vi "PID_Tuning.vi"() -> ()   [LabVIEW 2016]
uses:
  Classes/MotorControl/TypeDef/ControllerMode.ctl
  Classes/MotorControl/TypeDef/MotorTuneParam.ctl
  Classes/MotorControl/TypeDef/PID Param.ctl
  Classes/MotorControl/MotorControl.lvclass
  Classes/MotorControl/MotorControl.lvclass/MotorControl.ctl
  Classes/DataLogger/Data Logger.lvclass
  <vilib>/Platform/TimedLoop/XDataNode/timing_clust.ctl
  <vilib>/Platform/TimedLoop/XDataNode/nitl_modes.ctl
  <vilib>/Platform/TimedLoop/XDataNode/wakeup.ctl
  Classes/MotorControl/PropertyNodes/Motor_Read_Nx0.vi
  <vilib>/DAQmx/write.llb/DAQmx Write (Digital Bool 1Line 1Point).vi
  <vilib>/DAQmx/read.llb/DAQmx Read (Analog 1D Wfm NChan NSamp).vi
  <vilib>/Analysis/baseanly.llb/Mean (DBL).vi
  <vilib>/DAQmx/read.llb/DAQmx Read (Counter DBL 1Chan 1Samp).vi
  <vilib>/DAQmx/create/channels.llb/DAQmx Create Channel (CI-Position-Angular Encoder).vi
  <vilib>/FPGAPlugInAG/PXI-7842R/niLvFpga_Open_PXI-7842R.vi
  <vilib>/rvi/interface/common/dynamic/niFpgaDynamicAddResources.vi
  <vilib>/FPGAPlugInAG/Dynamic/niLvFpga_Reset_Dynamic.vi
  <vilib>/FPGAPlugInAG/Dynamic/niLvFpga_Run_Dynamic.vi
  <vilib>/Utility/error.llb/Error Cluster From Error Code.vi
  <vilib>/rvi/errors/niLvFpgaAdjustHostInterfaceError.vi
  GlobalVariables/Path_GV.vi
  <vilib>/DAQmx/miscellaneous.llb/DAQmx Fill In Error Info.vi
  <vilib>/measure/macond.llb/IIR Filter for N Chan.vi
  <vilib>/FPGAPlugInAG/Dynamic/niLvFpga_Close_Dynamic.vi
  <vilib>/rvi/interface/nirviOpenFPGA/nirviOpenFPGA.xnode
  FPGA Bitfiles/CAlex2_FPGATarget_MotorControl_+dy1qhm6Ymw.lvbitx
  FPGA/MotorControl_PWM+AO.vi
  <vilib>/rvi/interface/nirviMethod/nirviMethod.xnode
  <vilib>/rvi/interface/nirviReadWriteControl/nirviReadWriteControl.xnode
  <vilib>/Platform/TimedLoop/XDataNode/XDataNode.xnode
  <vilib>/rvi/interface/nirviCloseFPGA/nirviCloseFPGA.xnode
  <vilib>/Platform/TimedLoop/XDataNode/XDNodeRunTimeDep.lvlib
  <vilib>/rvi/interface/Simulation/niFpgaSimulationCallBeginRW.vi
  <vilib>/ptbypt/NI_PtbyPt.lvlib
  <vilib>/measure/NI_MABase.lvlib
  NiFpgaLv.dll
  <vilib>/Analysis/NI_AALBase.lvlib
  <vilib>/measure/NI_MAPro.lvlib
panel:
  out "MTP Changed":bool
  in  "Refresh List":bool
  in  "Set MTP":bool
  in  "Reset MTP":bool
  in  "Save MTP":bool
  in  "Load MTP":bool
  in  "Save MTP File":string
  in  "Motor Tuning Files":i32(listbox)
  in  "Motor Tuning Param":T1={"Transfer Ratio"=1.0, "Encoder CPR"=1000.0, "FeedForward Gain"=0.0, "FrictionParam"={"Coeff-Pos"=[0.0], "Coeff-Neg"=[0.0]}, "Force Rate"={"High"=10000.0, "Low"=100.0}, "PID Param"={"Setpoint Range"={"High"=100.0, "Low"=0.0}, "Output Range"={"High"=100.0, "Low"=-100.0}, "GainSchedules"=[{"PID gains"={"Kc"=1.0, "Ti"=0.0, "Td"=0.0}, "max value"=100.0}], "beta"=1.0, "gamma"=1.0, "linearity"=1.0}}
  in  "Input Mode":enum16{"Manual", "Func Gen", "Chirp"}(ring)
  in  "Offset":dbl=20.0
  in  "Magnitude":dbl=15.0
  out "Chirp Signal":dbl
  in  "Go Chirp":bool
  in  "Time":dbl
  in  "Freq High":dbl
  in  "Freq Low":dbl
  out "ShaftSpeed":dbl[](array[numeric])
  in  "decoding type":i32(ring)=10092 items=["X1"=10090, "X2"=10091, "X4"=10092, "Two Pulse Counting"=10313]
  in  "units":i32(ring)=10273 items=["Degrees"=10146, "Radians"=10273, "Ticks"=10304, "From Custom Scale"=10065]
  in  "pulses per revolution":u32=2048
  out "ShaftAngle":dbl[](array[numeric])
  in  "Tension Input IIR filter specifications":T3={"Topology"=enum."Off", "Type"=enum."Lowpass", "Order"=1, "Lower Fc"=100.0, "Upper Fc"=200.0, "PB Ripple"=1.0, "SB Attenuation"=60.0} {"PB Ripple" format="%0.2f"; "SB Attenuation" format="%0.2f"; "Lower Fc" format="%0.2p"; "Upper Fc" format="%0.2p"}
  out "Current Gain":i32
  out "PID Volt":dbl[](array[numeric])
  out "FF Volt":dbl[](array[numeric])
  in  "Softload? (T)":bool=TRUE
  in  "File Name":string
  in  "ProjectFolder":string="MotorTune"
  in  "Save":bool
  in  "Motor Mode":T4
  in  "LoadCell#":enum16{"1", "2", "3", "4", "5", "6", "7", "8"}(ring)
  in  "Manual Tension":dbl
  out "funcgen":dbl
  in  "reset signal":bool
  out "Signal Command":cluster{"upper limit":dbl}(graph)
  in  "Motor#":enum16{"1", "2", "3", "4", "5", "6", "7", "8"}(ring)
  in  "phase":dbl format="%.2p"
  in  "offset":dbl format="%0.2p"
  in  "signal type":T5(ring)
  in  "frequency":dbl=1.0 format="%0.2p"
  in  "amplitude":dbl=1.0 format="%0.2p"
  out "Max Duration":dbl format="%0.2f"
  in  "Friction Compensation(T)":bool=TRUE
  in  "Reinitialize? (F)":bool
  out "Voltage":sgl(graph)
  out "Tension":cluster{"[0]":dbl, "[1]":dbl}(graph)
  out "PlannedTension":dbl[](array[numeric])
  in  "stop":bool
  out "PID Duration":dbl
  out "Actual Tensions":dbl[](array[numeric])
  out "Fric Volt":dbl[](array[numeric])
  out "AO_Value":sgl[](array[numeric])
  in  "Enabled":bool[](array[boolean])=[FALSE, FALSE, FALSE, FALSE, FALSE, FALSE, FALSE, FALSE]
  # "beta specifies the relative emphasis of setpoint tracking to disturbance rejection. The default value of 1 is appropriate for most applications. You can use a smaller value between 0 and 1 to specify emphasis on disturbance rejection, such as process load changes. The VI uses this value in the two degree-of-freedom algorithm."
  # "linearity specifies the linearity of the error response. The valid range for linearity is 0 to 1. A value of 1 provides a normal linear response, while a value of 0.1 provides an approximately parabolic response. The VI uses this value in the nonlinear error calculation and the nonlinear gain factor calculation."
  # "gamma specifies an amount by which to weight the error applied to derivative action. The default value is 0, which avoids the derivative kick, or sudden change in controller output, that can occur after a change in the setpoint value.\n\nIn certain cascade control operations where derivative kick is not a concern, increasing gamma might improve the speed of the first PID controller."
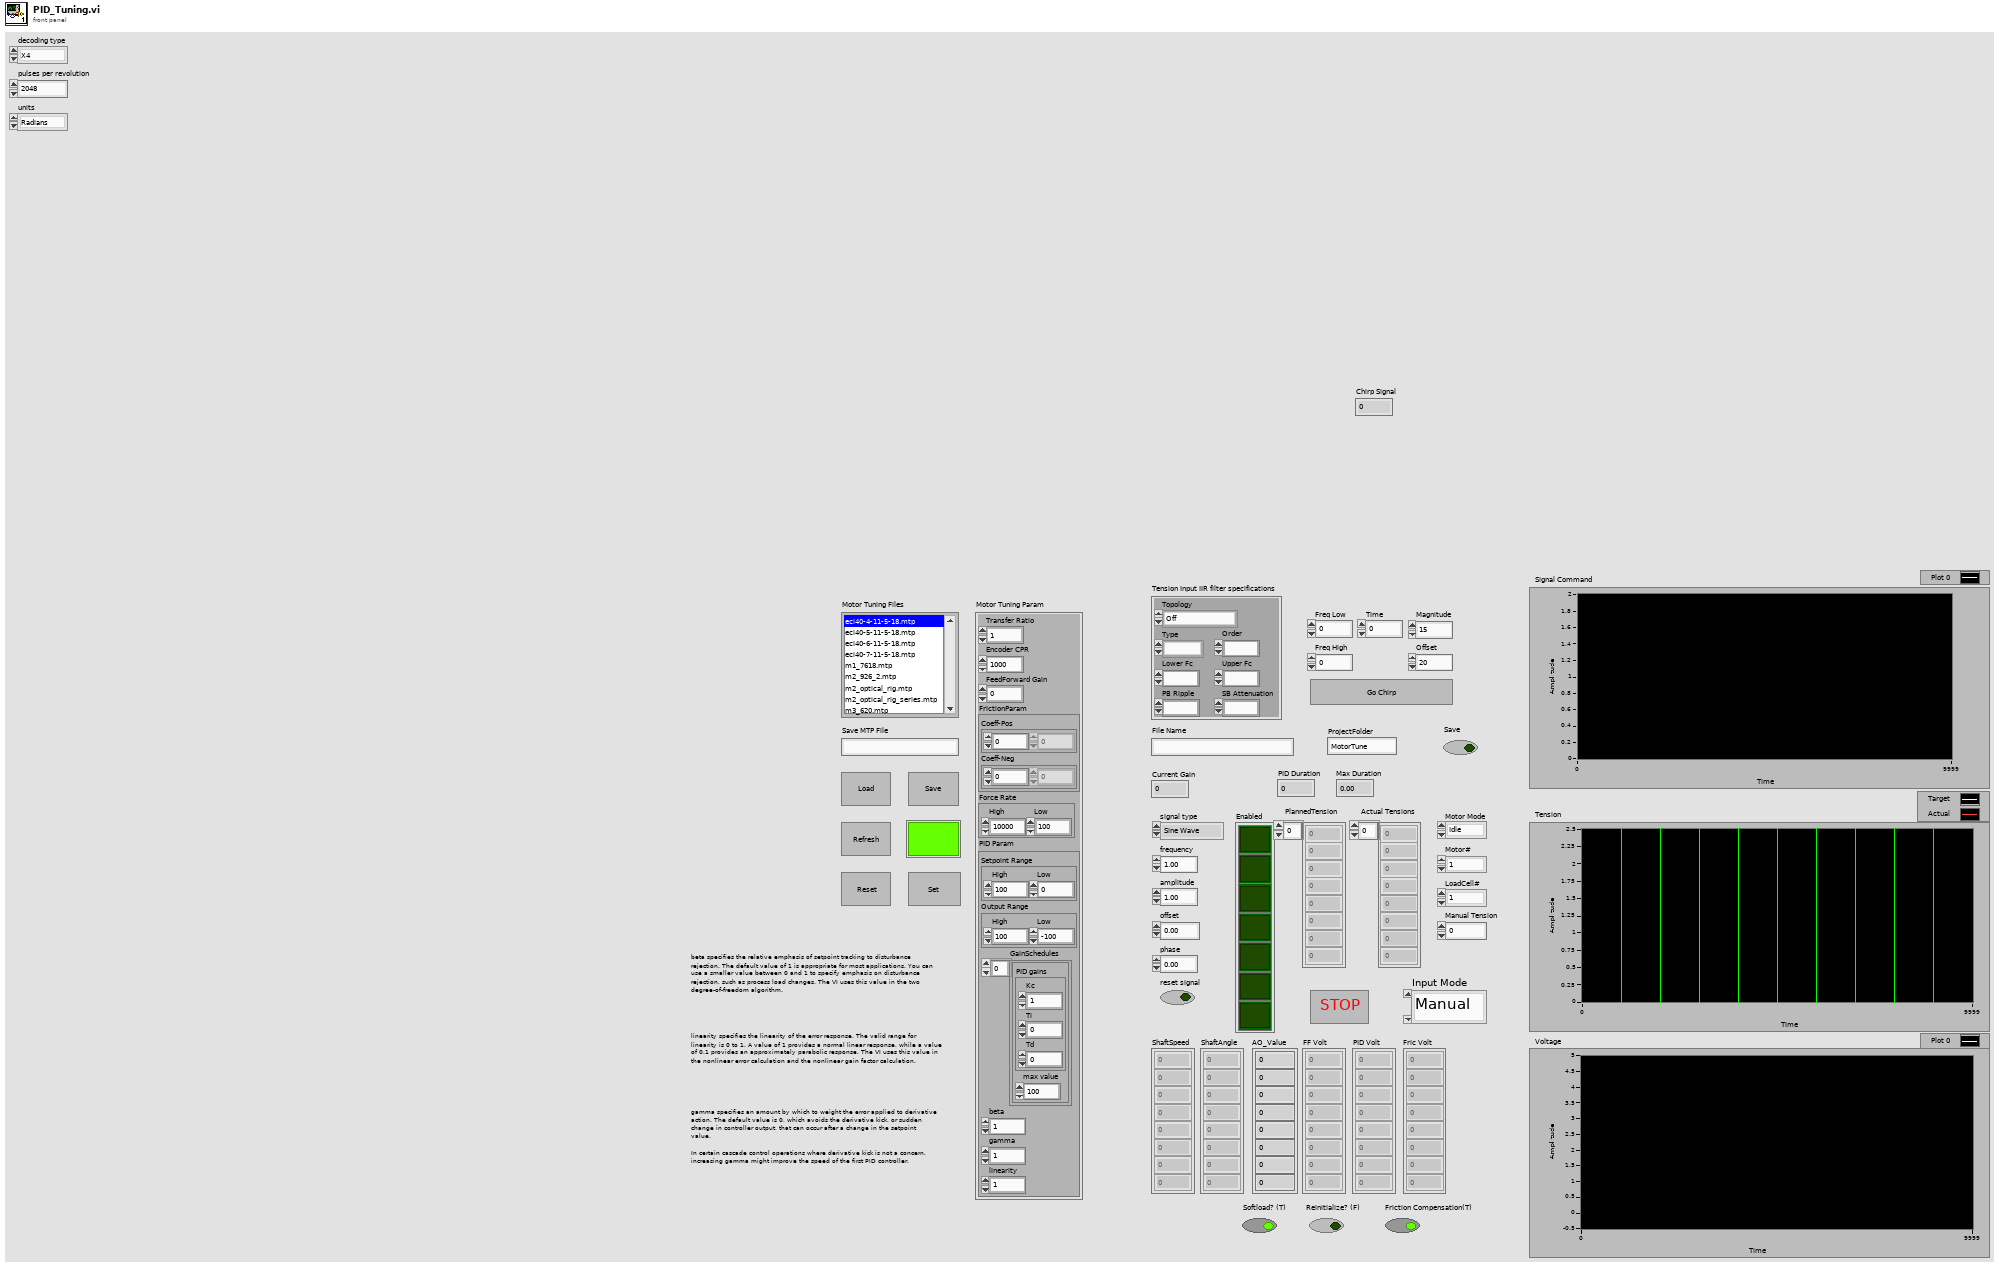
[diagram p1: front panel]
types:
  T1 = typedef "MotorControl.lvclass/MotorTuneParam.ctl" = cluster{"Transfer Ratio":dbl, "Encoder CPR":dbl, "FeedForward Gain":dbl, "FrictionParam":cluster{"Coeff-Pos":dbl[], "Coeff-Neg":dbl[]}, "Force Rate":cluster{"High":dbl, "Low":dbl}, "PID Param":T2}
  T2 = typedef "MotorControl.lvclass/PID Param.ctl" = cluster{"Setpoint Range":cluster{"High":dbl, "Low":dbl}, "Output Range":cluster{"High":dbl, "Low":dbl}, "GainSchedules":cluster{"PID gains":cluster{"Kc":dbl, "Ti":dbl, "Td":dbl}, "max value":dbl}[], "beta":dbl, "gamma":dbl, "linearity":dbl}
  T3 = cluster{"Topology":enum16{"Off", "Butterworth", "Chebyshev", "Inverse Chebyshev", "Elliptic", "Bessel"}, "Type":enum16{"Lowpass", "Highpass", "Bandpass", "Bandstop"}, "Order":i32, "Lower Fc":dbl, "Upper Fc":dbl, "PB Ripple":dbl, "SB Attenuation":dbl}
  T4 = typedef "MotorControl.lvclass/ControllerMode.ctl" = enum16{"Idle", "FF", "PID"}
  T5 = enum16{"Sine Wave", "Triangle Wave", "Square Wave", "Sawtooth Wave"}
  T6 = typedef "XDNodeRunTimeDep.lvlib/timing_clust.ctl" = cluster{"Expected End [f-1]":u64, "Actual End [f-1]":u64, "Finished Late? [f-1]":bool, "Expected End [i-1]":u64, "Actual End [i-1]":u64, "Finished Late? [i-1]":bool, "Expected Start [i]":u64, "Actual Start [i]":u64, "Expected Start [f]":u64, "Actual Start [f]":u64, "Source Name":string, "Structure Name":string, "Period":i64, "Deadline":i64, "Offset":i64, "Start":i64, "Priority":i32, "Timeout":i32, "Mode":T7, "Wakeup Reason":T8, "Error":errorcluster, "Source Type":string, "Secondary Source Type":string, "Global End Time":u64, "Global Start Time":u64, "Frame Duration":u64, "Iteration Duration":u64, "Assigned CPU":i32, "I/O Scan Engine Mode":u32}
  T7 = typedef "XDNodeRunTimeDep.lvlib/nitl_modes.ctl" = enum32{"No Change", "Process missed periods, maintain original phase", "Discard missed periods, maintain original phase", "Process missed periods, ignore original phase", "Discard missed periods, ignore original phase"}
  T8 = typedef "XDNodeRunTimeDep.lvlib/wakeup.ctl" = enum32{"Normal", "Aborted", "Asynchronous wakeup", "Timing source error", "Timed loop error", "Timeout"}
  T9 = cluster{"FF Vol":dbl[], "Filtered PID":dbl[], "Fric Volatage":dbl[], "Unfiltered PID":dbl[]}
  T10 = cluster{"PID gains":cluster{"Kc":dbl, "Ti":dbl, "Td":dbl}, "max value":dbl}[]
  T11 = cluster{"PID gains":cluster{"Kc":dbl, "Ti":dbl, "Td":dbl}, "max value":dbl}
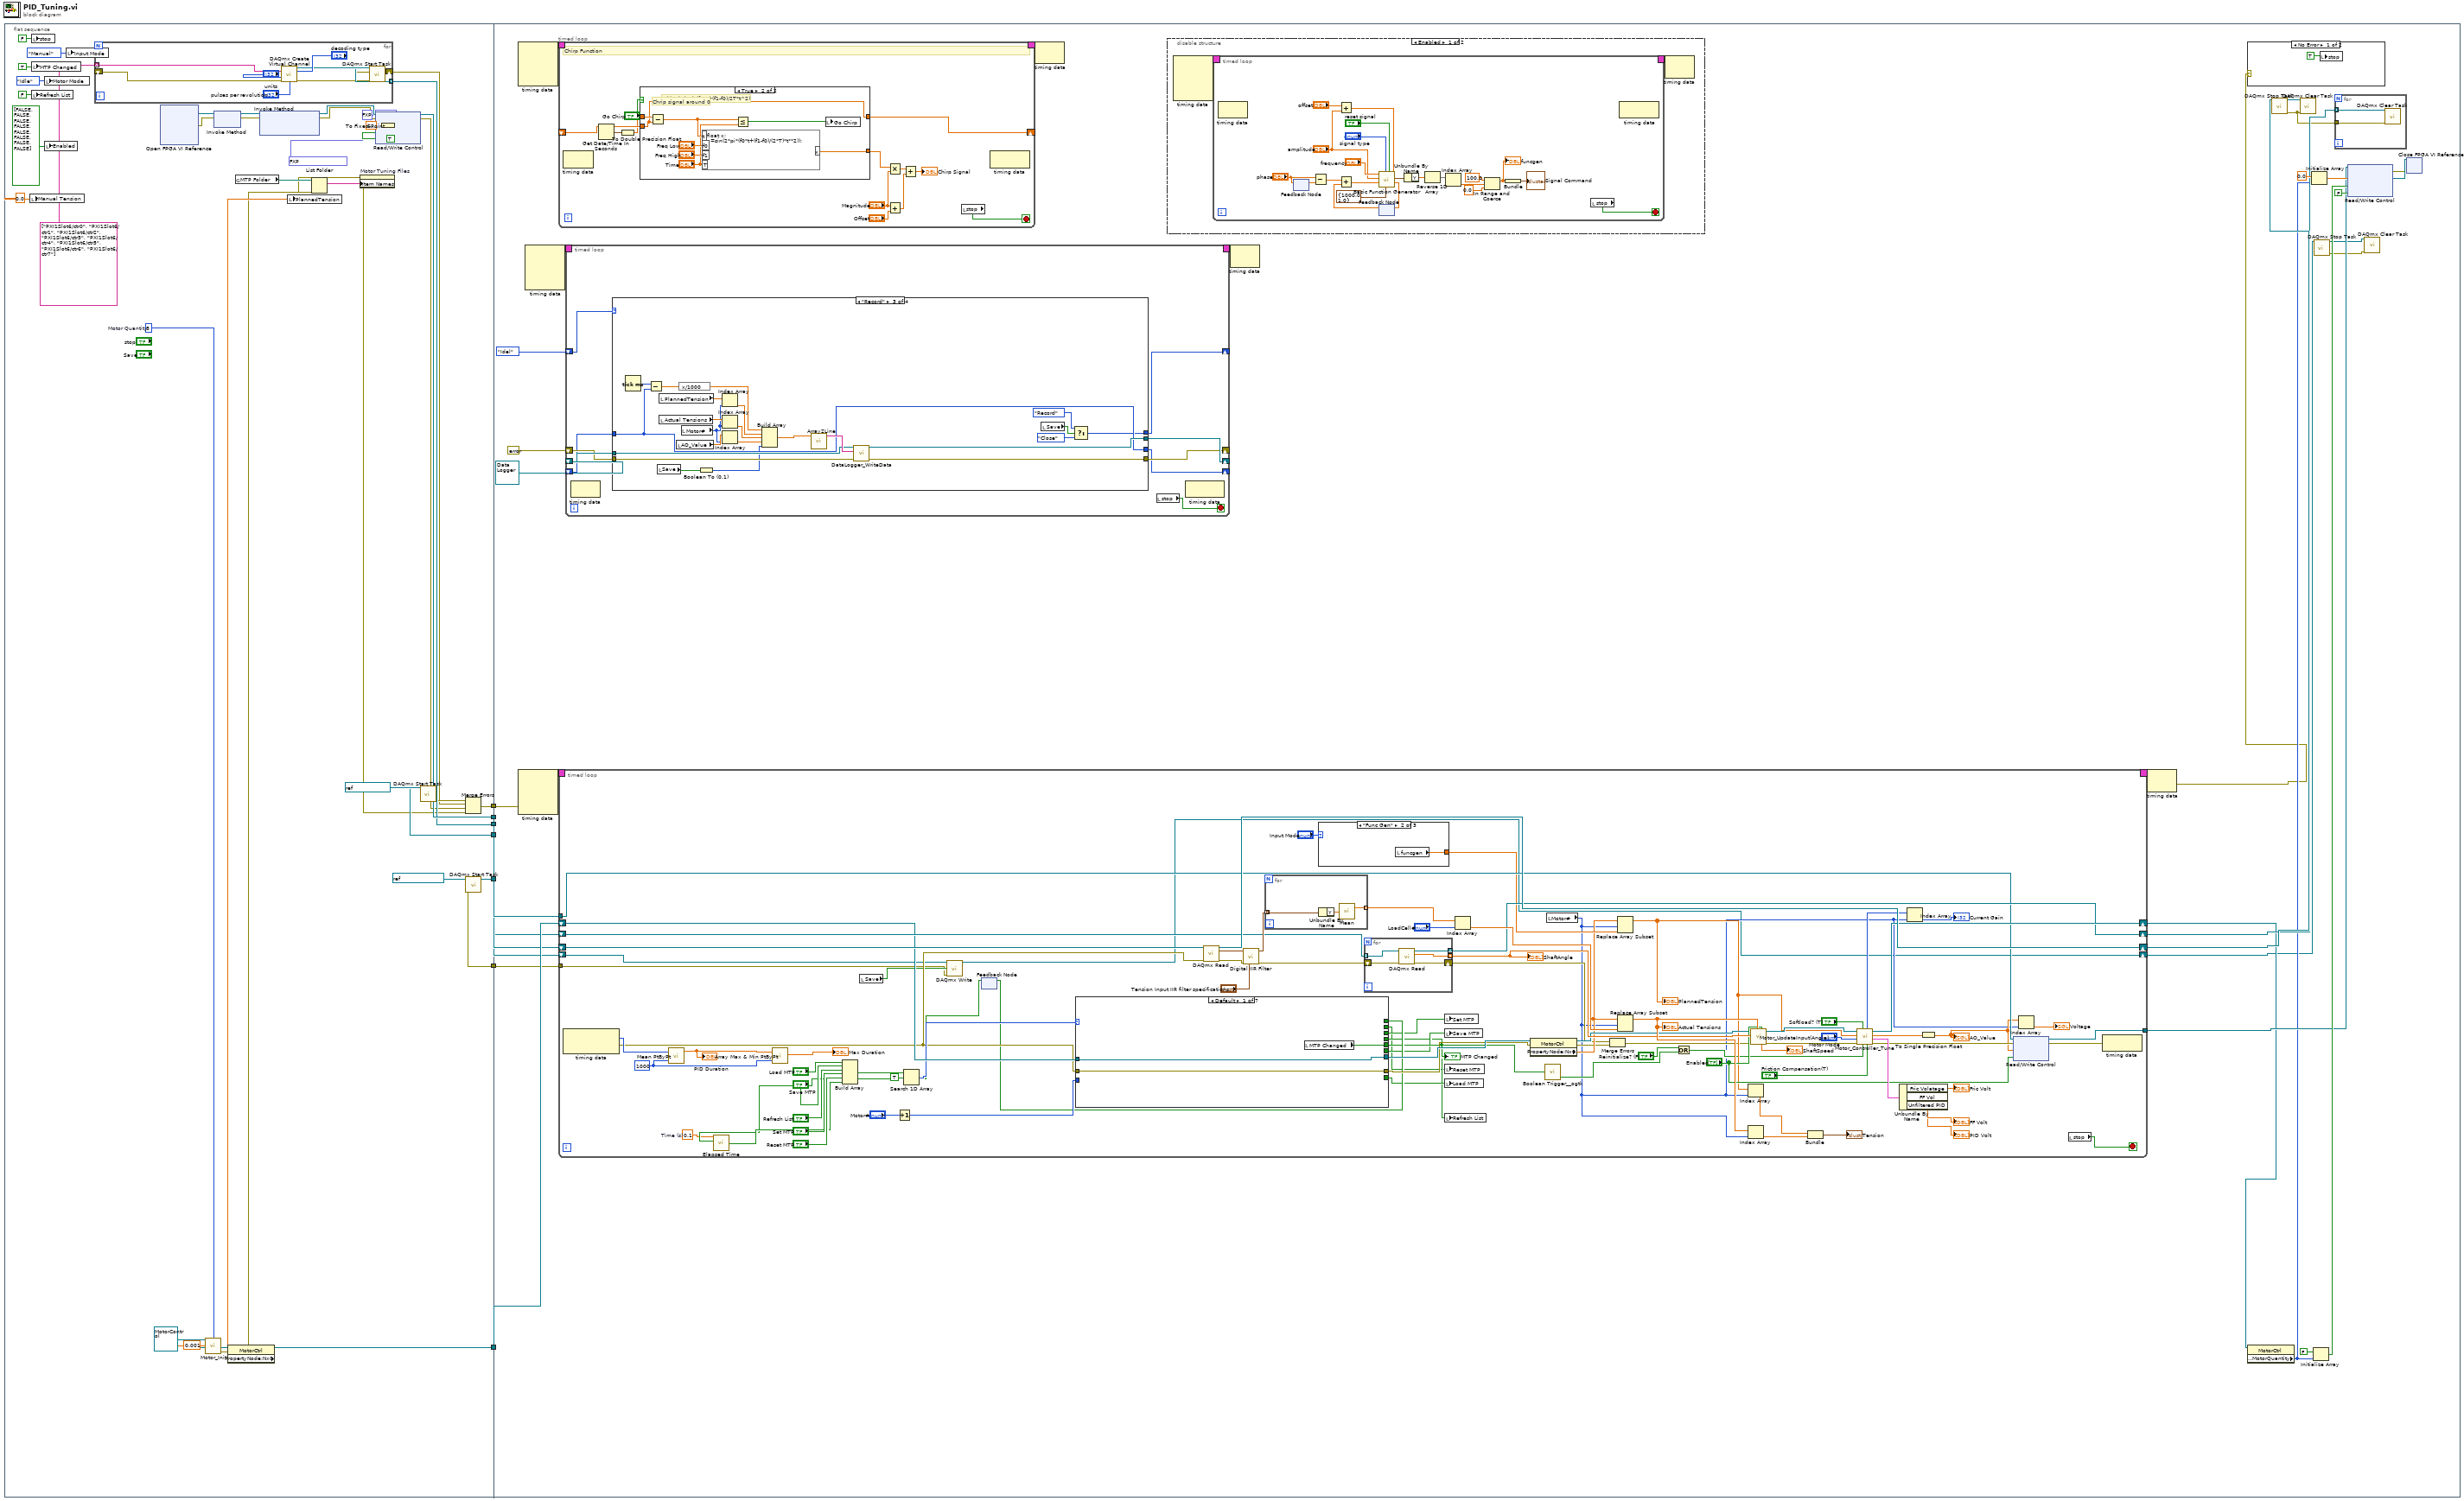
[diagram p0: block diagram]
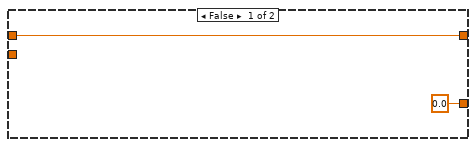
[diagram p3: hidden frame]
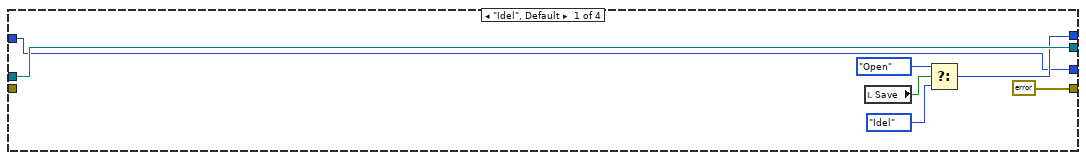
[diagram p4: hidden frame]
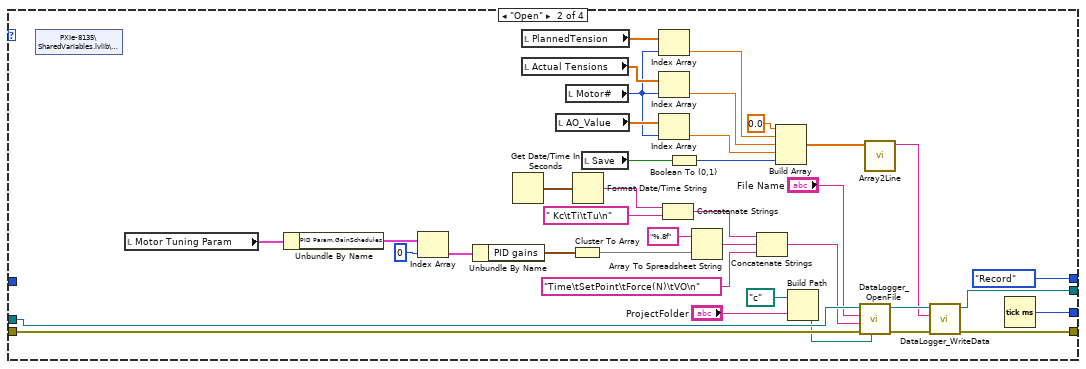
[diagram p5: hidden frame]
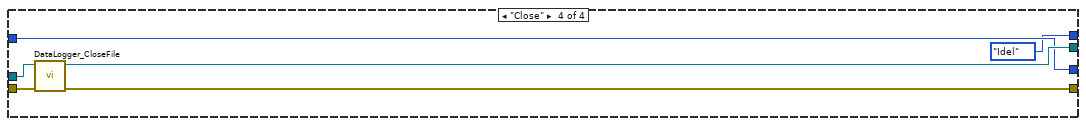
[diagram p6: hidden frame]
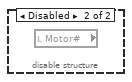
[diagram p7: hidden frame]
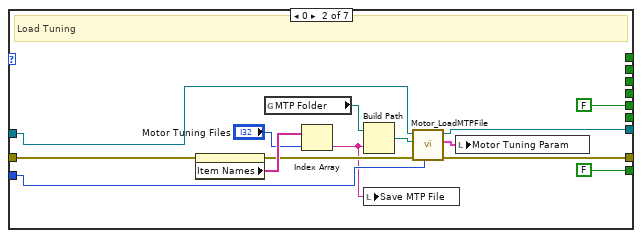
[diagram p8: hidden frame]
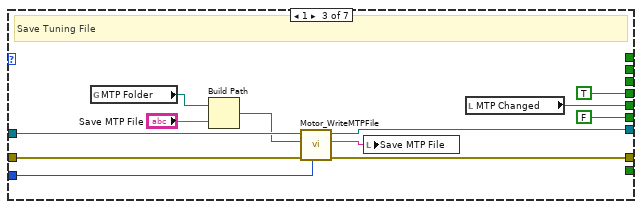
[diagram p9: hidden frame]
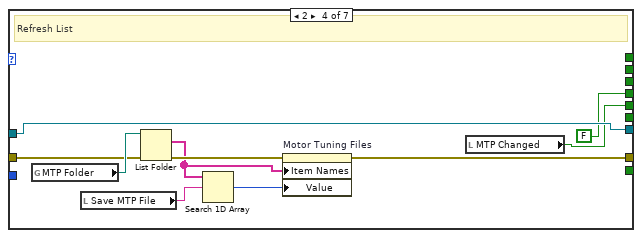
[diagram p10: hidden frame]
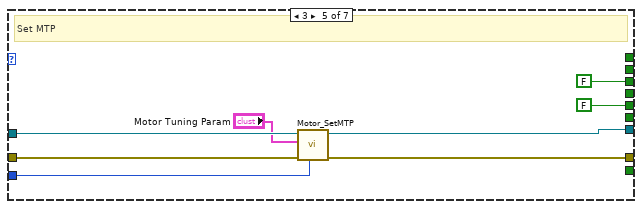
[diagram p11: hidden frame]
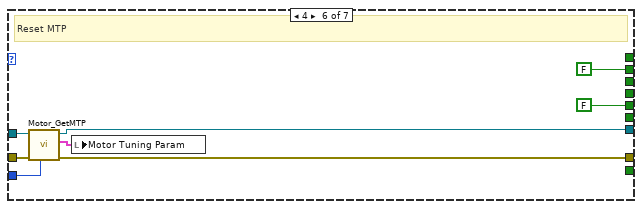
[diagram p12: hidden frame]
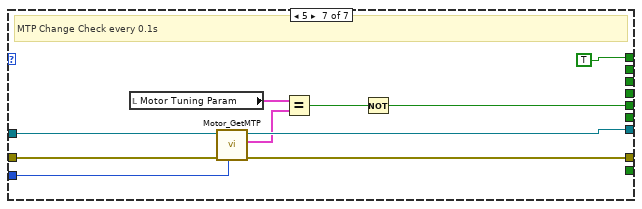
[diagram p13: hidden frame]
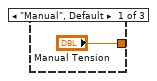
[diagram p14: hidden frame]
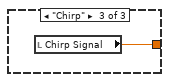
[diagram p15: hidden frame]
diagram:
  n1 = flat-sequence {
    tunnel: [w41] -> w7
    tunnel: [w17] -> w6
    tunnel: [w34] -> w5
    tunnel: [w32] -> w4
    tunnel: [w30] -> w3
    tunnel: [w9] -> w2
    tunnel: [w8] -> w1
    tunnel: w7 -> [w90]
    tunnel: w6 -> [w89]
    tunnel: w5 -> [w88]
    tunnel: w4 -> [w73]
    tunnel: w3 -> [w68]
    tunnel: w2 -> [w63]
    tunnel: w1 -> [w62]
    frame #0 {
      w13 = 8  # Motor Quantity
      n2 = local write "Manual Tension"(0.0 ("Planned Tension")) -> ()
      n3 = local write "stop"(FALSE ("stop")) -> ()
      n4 = local write "MTP Changed"(TRUE ("MTP Changed")) -> ()
      n5 = local write "Refresh List"(FALSE ("Refresh List")) -> ()
      n6 = local write "Motor Mode"(ControllerMode."Idle" ("Mode")) -> ()
      n7 = local write "Enabled"(bool[] [FALSE, FALSE, FALSE, FALSE, FALSE, FALSE, FALSE, FALSE] ("Enabled")) -> ()
      n8 = local write "Input Mode"(enum16{"Manual", "Func Gen", "Chirp"}."Manual" ("Input Mode")) -> ()
      n9 = for {
        tunnel: tag[] ["PXI1Slot6/ctr0", "PXI1Slot6/ctr1", "PXI1Slot6/ctr2", "PXI1Slot6/ctr3", "PXI1Slot6/ctr4", "PXI1Slot6/ctr5", "PXI1Slot6/ctr6", "PXI1Slot6/ctr7"] ("Encoder Tasks In") -> [w58] mode=indexing
        tunnel: [w52] -> w32 mode=indexing
        shift-right: [w50] -> w28
        shift-left: _ -> [w55]
        n10 = call-poly <vilib>:"DAQmx Create Virtual Channel.vi"("counter"=w58, "decoding type"="decoding type", "units"="units", "error in"=w55, "pulses per revolution"="pulses per revolution") -> ("task out"=w53:refnum<k21>, "error out"=w51:errorcluster)  [unwired: 9 in]
        n11 = call <vilib>:"DAQmx Start Task.vi"("task/channels in"=w53, "error in"=w51) -> ("task out"=w52:refnum<k21>, "error out"=w50:errorcluster)  [unwired: 12 in]
      }
      n12 = xnode "Open FPGA VI Reference"() -> ("FPGA VI Reference Out"=w42:refnum<k20>, "error out"=w45:errorcluster)  [unwired: 2 in]
      n13 = call "Motor_Init.vi"("Motor Control In"=refnum<class "MotorControl.lvclass"> refnum, "Motor Quantity(1)"=w13, "PID Loop Period(0.001)"=0.001 ("PID Loop Period")) -> ("Motor Control Out"=w15:refnum<class "MotorControl.lvclass">, "error out"=w14:errorcluster)  [unwired: 11 in]
      n14 = xnode "Invoke Method"("FPGA VI Reference In"=w42, "error in"=w45) -> ("FPGA VI Reference Out"=w43:refnum<k20>, "error out"=w44:errorcluster)
      n15 = property class="MotorCtrl"(reference=w15, error in=w14) -> (reference out=w17:refnum<class "MotorControl.lvclass">, error out=w18:errorcluster, "PropertyNode:Nx0"=w19:dbl[])
      n16 = global read "Path_GV.vi" "MTP Folder"() -> (w23:path)
      n17 = xnode "Invoke Method"("FPGA VI Reference In"=w43, "error in"=w44) -> ("FPGA VI Reference Out"=w49:refnum<k20>, "error out"=w40:errorcluster)  [unwired: 1 in]
      n18 = local write "PlannedTension"(w19) -> ()
      n19 = List Folder(path=w23, error in=w18) -> (filenames=w24:string[], error out=w21:errorcluster)  [unwired: 2 in, 2 out]
      n20 = property on="Motor Tuning Files" class="LstBox (strict)"(error in=w21, "Item Names"=w24) -> (error out=w25:errorcluster)  [unwired: 1 in, 1 out]
      n21 = To Fixed-Point(fixed-point type=fxp<+/-,32,10> 0.0 ("2pi"), number=6.283185307179586) -> (fixed-point=w47:fxp<+/-,32,10>)
      n22 = xnode "Read/Write Control"("FPGA VI Reference In"=w49, "error in"=w40, "2pi"=w47, "EnableMaster"=TRUE, "PWM (Hz/A)"=fxp<+/-,32,16> 13.333328247070312) -> ("FPGA VI Reference Out"=w41:refnum<k20>, "error out"=w27:errorcluster)
      n23 = call <vilib>:"DAQmx Start Task.vi"("task/channels in"=refnum<k21> "TuningTask" ("Analog Input Channels")) -> ("task out"=w34:refnum<k21>, "error out"=w29:errorcluster)  [unwired: 13 in]
      n24 = Merge Errors(w29, w28, w27, w25) -> (w30:errorcluster)
      n25 = call <vilib>:"DAQmx Start Task.vi"("task/channels in"=refnum<k21> "SyncOut_EMG" ("DAQmx Task Name")) -> ("task out"=w9:refnum<k21>, "error out"=w8:errorcluster)  [unwired: 13 in]
    }
    frame #1 {
      n26 = node-c288() -> (w70:T6)  [unwired: 4 in]
      n27 = node-c288(w68) -> (w92:T6)  [unwired: 3 in]
      n28 = node-c288() -> (w80:T6)  [unwired: 4 in]
      n29 = timed-loop {
        timing: w70 -> [_]
        timing-out: [_] -> w69
        shift-right: [w104] -> _
        shift-left: _ -> [w103]
        stop <- w105 stop-if-true
        # "x(t)=sin(2pi*(f0*t+(f1-f0)/2T*t^2)"
        # "Chirp Function"
        n30 = node-c288() -> ()  [unwired: 1 in, 1 out]
        n31 = Get Date/Time In Seconds() -> (seconds since 1Jan1904=w101:timestamp)
        n32 = To Double Precision Float(number=w101) -> (double precision float=w100:dbl)
        n33 = case shown="True" "Go Chirp" {
          tunnel: [w107 w109] -> w104
          tunnel: w103 -> [_ w109]
          tunnel: [0.0 w108] -> w96
          tunnel: w100 -> [w107 w113]
          frame False {
          }
          frame True {
            # "Chrip signal around 0"
            n34 = Subtract(x=w113, y=w109) -> (x-y=w112:dbl)
            n35 = formula code="float x;\nx=sin(2*pi*(f0*t+(f1-f0)/(2*T)*t**2));"("t"=w112, "f0"="Freq Low", "f1"="Freq High", "T"="Time") -> ("x"=w108:dbl)
            n36 = Less Or Equal?(x=w112, y="Time") -> (x <= y?=w110:bool)
            n37 = local write "Go Chirp"(w110) -> ()
          }
        }
        n38 = Multiply(x=w96, y="Magnitude") -> (x*y=w97:dbl)
        n39 = Add(x="Magnitude", y="Offset") -> (x+y=w98:dbl)
        n40 = Add(x=w97, y=w98) -> (x+y=→"Chirp Signal":dbl)
        n41 = local read "stop"() -> (w105:bool)
        n42 = node-c288() -> ()  [unwired: 1 in, 1 out]
      }
      n43 = timed-loop {
        timing: w92 -> [_]
        timing-out: [_] -> w91
        shift-right: [w314] -> w66
        shift-left: w89 -> [w266]
        shift-right: [w318] -> w75
        shift-left: w88 -> [w319]
        tunnel: w90 -> [w290]
        tunnel: [w316] -> w67
        shift-right: [w293] -> w72
        shift-left: w73 -> [w294]
        shift-right: [w239] -> w59
        shift-left: w63 -> [w240]
        tunnel: w62 -> [w237]
        stop <- w317 stop-if-true
        w252 = 0.1  # Time (s)
        w311 = 1000 ("sample length")
        n44 = node-c288() -> (w313:i64, w263:errorcluster)  [unwired: 1 in]
        n45 = call <vilib>:"Mean PtByPt.vi"("x"=w313, "sample length"=w311) -> ("mean"=w312:dbl)  [unwired: 2 in, 1 out]
        "PID Duration" <- w312
        n46 = call <vilib>:"Array Max & Min PtByPt.vi"("input data point"=w312, "sample length"=w311) -> ("max value"=→"Max Duration":dbl)  [unwired: 1 in, 4 out]
        n47 = local read "Save"() -> (w238:bool)
        n48 = Increment(x="Motor#") -> (x+1=w261:enum16{"1", "2", "3", "4", "5", "6", "7", "8"})
        n49 = call-poly <vilib>:"DAQmx Write.vi"("task/channels in"=w240, "data"=w238, "error in"=w237) -> ("task out"=w239:refnum<k21>)  [unwired: 10 in, 2 out]
        n50 = feedback #1() -> (w253:bool)  [unwired: 1 in]
        n51 = call "Elapsed Time"("Time Target (s)"=w252, "Reset"=w253) -> ("Time has Elapsed"=w255:bool)  [unwired: 10 in, 7 out]
        n52 = Build Array("Load MTP", "Save MTP", "Refresh List", "Set MTP", "Reset MTP", w255) -> (w271:bool[])
        n53 = Search 1D Array(1D array=w271, element=TRUE) -> (index of element=w264:i32)  [unwired: 1 in]
        n54 = case shown="Default" w264 {
          tunnel: w266 -> [w322 w336 w348 w358 w366 w374 w384]
          tunnel: [w322 w335 w347 w358 w365 w373 w383] -> w265
          tunnel: w263 -> [w321 w330 w346 w354 w363 w371 w381]
          tunnel: [w321 w334 w345 w356 w364 w372 w382] -> w262
          tunnel: w261 -> [_ w326 w340 _ w361 w370 w380]
          tunnel: [_ _ _ _ _ _ TRUE] -> w254
          tunnel: [w320 FALSE ("MTP Changed") w339 w353 FALSE ("MTP Changed") FALSE ("MTP Changed") w375] -> w249
          tunnel: [_ FALSE ("Load MTP") _ _ _ _ _] -> w246
          tunnel: [_ _ FALSE ("Save MTP") _ _ _ _] -> w245
          tunnel: [_ _ TRUE ("Refresh List") FALSE ("Refresh List") _ _ _] -> w244
          tunnel: [_ _ _ _ FALSE ("Set MTP") _ _] -> w243
          tunnel: [_ _ _ _ _ FALSE ("Reset MTP") _] -> w242
          frame Default {
            n55 = local read "MTP Changed"() -> (w320:bool)
          }
          frame 0 {
            # "Load Tuning"
            n56 = property on="Motor Tuning Files" class="LstBox (strict)"(error in=w330) -> (error out=w329:errorcluster, "Item Names"=w331:string[])  [unwired: 1 in, 1 out]
            n57 = global read "Path_GV.vi" "MTP Folder"() -> (w332:path)
            n58 = Index Array(array=w331, index="Motor Tuning Files") -> (element=w323:string)
            n59 = Build Path(base path=w332, name or relative path=w323) -> (appended path=w328:path)
            n60 = local write "Save MTP File"(w323) -> ()
            n61 = call "Motor_LoadMTPFile.vi"("Motor ID (1-indexed)"=w326, "error in (no error)"=w329, "Tuning Files Path"=w328, "MotorCtrl in"=w336) -> ("error out"=w334:errorcluster, "MTP Data (dup)"=w333:T1, "MotorCtrl out"=w335:refnum<class "MotorControl.lvclass">)  [unwired: 5 in]
            n62 = local write "Motor Tuning Param"(w333) -> ()
          }
          frame 1 {
            # "Save Tuning File"
            n63 = global read "Path_GV.vi" "MTP Folder"() -> (w344:path)
            n64 = Build Path(base path=w344, name or relative path="Save MTP File") -> (appended path=w342:path)
            n65 = call "Motor_WriteMTPFile.vi"("Motor ID (1-indexed)"=w340, "error in (no error)"=w346, "Save Path"=w342, "MotorCtrl in"=w348) -> ("error out"=w345:errorcluster, "Actual File Name"=w341:string, "MotorCtrl out"=w347:refnum<class "MotorControl.lvclass">)  [unwired: 5 in]
            n66 = local write "Save MTP File"(w341) -> ()
            n67 = local read "MTP Changed"() -> (w339:bool)
          }
          frame 2 {
            # "Refresh List"
            n68 = global read "Path_GV.vi" "MTP Folder"() -> (w357:path)
            n69 = local read "Save MTP File"() -> (w350:string)
            n70 = List Folder(path=w357, error in=w354) -> (filenames=w351:string[], error out=w355:errorcluster)  [unwired: 2 in, 2 out]
            n71 = Search 1D Array(1D array=w351, element=w350) -> (index of element=w349:i32)  [unwired: 1 in]
            n72 = property on="Motor Tuning Files" class="LstBox (strict)"(error in=w355, "Item Names"=w351, "Value"=w349) -> (error out=w356:errorcluster)  [unwired: 1 in, 1 out]
            n73 = local read "MTP Changed"() -> (w353:bool)
          }
          frame 3 {
            # "Set MTP"
            n74 = call "Motor_SetMTP.vi"("Motor ID (1-indexed)"=w361, "error in (no error)"=w363, "Motor Tuning Param"="Motor Tuning Param", "MotorCtrl in"=w366) -> ("error out"=w364:errorcluster, "MotorCtrl out"=w365:refnum<class "MotorControl.lvclass">)  [unwired: 6 in]
          }
          frame 4 {
            # "Reset MTP"
            n75 = call "Motor_GetMTP.vi"("Motor ID (1-indexed)"=w370, "error in (no error)"=w371, "MotorCtrl in"=w374) -> ("error out"=w372:errorcluster, "Motor Tuning Param"=w369:T1, "MotorCtrl out"=w373:refnum<class "MotorControl.lvclass">)  [unwired: 6 in]
            n76 = local write "Motor Tuning Param"(w369) -> ()
          }
          frame 5 {
            # "MTP Change Check every 0.1s"
            n77 = local read "Motor Tuning Param"() -> (w379:T1)
            n78 = call "Motor_GetMTP.vi"("Motor ID (1-indexed)"=w380, "error in (no error)"=w381, "MotorCtrl in"=w384) -> ("error out"=w382:errorcluster, "Motor Tuning Param"=w378:T1, "MotorCtrl out"=w383:refnum<class "MotorControl.lvclass">)  [unwired: 6 in]
            n79 = Equal?(x=w379, y=w378) -> (x = y?=w376:bool)
            n80 = Not(x=w376) -> (.not. x?=w375:bool)
          }
        }
        "MTP Changed" <- w249
        n81 = feedback-in #1(w254) -> ()
        n82 = call-poly <vilib>:"DAQmx Read.vi"("task/channels in"=w319, "error in"=w263) -> ("task out"=w318:refnum<k21>, "data"=w298:waveform(dbl)[], "error out"=w274:errorcluster)  [unwired: 11 in]
        n83 = call-poly <vilib>:"Digital IIR Filter.vi"("IIR filter specifications"="Tension Input IIR filter specifications", "error in (no error)"=w274, "signal(s) in"=w298) -> ("error out"=w273:errorcluster, "signal(s) out"=w297:waveform(dbl)[])  [unwired: 6 in, 1 out]
        n84 = for {
          tunnel: w297 -> [w395] mode=indexing
          tunnel: [w393] -> w296 mode=indexing
          n85 = Unbundle By Name(w395) -> ("Y"=w394:dbl[])
          n86 = call-poly <vilib>:"Mean.vi"("X"=w394) -> ("mean"=w393:dbl)  [unwired: 1 out]
        }
        n87 = case shown="\"Func Gen\"" "Input Mode" {
          tunnel: ["Manual Tension" w386 w387] -> w288
          frame "Manual", Default {
          }
          frame "Func Gen" {
            n88 = local read "funcgen"() -> (w386:dbl)
          }
          frame "Chirp" {
            n89 = local read "Chirp Signal"() -> (w387:dbl)
          }
        }
        n90 = for {
          tunnel: w294 -> [w389] mode=indexing
          tunnel: [w392] -> w291 mode=indexing
          tunnel: [w391] -> w293 mode=indexing
          shift-right: [w390] -> w258
          shift-left: w273 -> [w388]
          n91 = call-poly <vilib>:"DAQmx Read.vi"("task/channels in"=w389, "error in"=w388) -> ("task out"=w391:refnum<k21>, "data"=w392:dbl, "error out"=w390:errorcluster)  [unwired: 11 in]
        }
        "ShaftAngle" <- w291
        n92 = local write "Set MTP"(w243) -> ()
        n93 = local write "Save MTP"(w245) -> ()
        n94 = local write "Reset MTP"(w242) -> ()
        n95 = local write "Load MTP"(w246) -> ()
        n96 = local write "Refresh List"(w244) -> ()
        n97 = Index Array(array=w296, index="LoadCell#") -> (element=w309:dbl)
        n98 = property class="MotorCtrl"(reference=w265, error in=w262) -> (reference out=w277:refnum<class "MotorControl.lvclass">, error out=w257:errorcluster, "PropertyNode:Nx0"=w260:dbl[])
        n99 = call <userlib>:"Boolean Trigger__ogtk.vi"("Boolean Input"=w249) -> ("Falling Edge"=w248:bool)  [unwired: 1 in, 1 out]
        n100 = local read "Motor#"() -> (w241:enum16{"1", "2", "3", "4", "5", "6", "7", "8"})
        n101 = Merge Errors(w258, w257) -> (w259:errorcluster)
        n102 = Replace Array Subset(array=w260, new element=w288, index=w241) -> (w275:dbl[])
        "PlannedTension" <- w275
        n103 = Replace Array Subset(array=w260, new element=w309, index=w241) -> (w301:dbl[])
        "Actual Tensions" <- w301
        n104 = Or(x="Reinitialize? (F)", y=w248) -> (x .or. y?=w250:bool)
        n105 = Index Array(array=w275, index=w241) -> (element=w282:dbl)
        n106 = Index Array(array=w301, index=w241) -> (element=w281:dbl)
        n107 = call "Motor_UpdateInput(Angle).vi"("Enabled"="Enabled", "CableTensionNow(N)"=w301, "error in (no error)"=w259, "MotorEncAngle(rad)"=w291, "Motor in"=w277) -> ("error out"=w285:errorcluster, "Motor out"=w286:refnum<class "MotorControl.lvclass">, "Angular Rate(rad/s)"=→"ShaftSpeed":dbl[])  [unwired: 3 in, 1 out]
        n108 = Bundle("Numeric"=w282, "Numeric"=w281) -> (→"Tension":cluster{"Numeric":dbl, "Numeric":dbl})  [unwired: 1 in]
        n109 = call "Motor_Controller_Tune.vi"("Friction Compensation(F)"="Friction Compensation(T)", "Reinitialize? (F)"=w250, "Softload? (T)"="Softload? (T)", "error in (no error)"=w285, "Mode"="Motor Mode", "CableTensionRef(N)"=w275, "Motor in"=w286) -> ("error out"=w280:errorcluster, "Detailed Voltage"=w305:T9, "VoltageCommand"=w284:dbl[], "Motor out"=w314:refnum<class "MotorControl.lvclass">, "PID Gain Idx"=w302:i32[])
        n110 = Unbundle By Name(w305) -> ("Fric Volatage"=→"Fric Volt":dbl[], "FF Vol"=→"FF Volt":dbl[], "Unfiltered PID"=→"PID Volt":dbl[])
        n111 = Index Array(array=w302, index=w241) -> (element=→"Current Gain":i32)
        n112 = To Single Precision Float(number=w284) -> (single precision float=w276:sgl[])
        "AO_Value" <- w276
        n113 = xnode "Read/Write Control"("FPGA VI Reference In"=w290, "error in"=w280, "AmpCmd"=w276, "Enable"="Enabled") -> ("FPGA VI Reference Out"=w316:refnum<k20>, "error out"=w279:errorcluster)
        n114 = Index Array(array=w276, index=w241) -> (element=→"Voltage":sgl)
        n115 = local read "stop"() -> (w317:bool)
        n116 = node-c288(w279) -> ()  [unwired: 1 out]
      }
      n117 = timed-loop {
        timing: w80 -> [_]
        timing-out: [_] -> w79
        shift-right: [w128] -> _
        shift-left: refnum<class "Data Logger.lvclass"> refnum ("Data Logger out") -> [w129]
        shift-right: [w127] -> _
        shift-left: errorcluster {"status"=FALSE, "code"=0, "source"=""} ("error out") -> [w126]
        shift-right: [w124] -> _
        shift-left: _ -> [w125]
        shift-right: [w123] -> _
        shift-left: enum16{"Close", "Record", "Open", "Idel"}."Idel" -> [w130]
        stop <- w122 stop-if-true
        n118 = node-c288() -> ()  [unwired: 1 in, 1 out]
        n119 = case shown="\"Record\"" w130 {
          tunnel: w129 -> [w137 w175 w194 w204]
          tunnel: [w137 w174 w198 w202] -> w128
          tunnel: [errorcluster {"status"=FALSE, "code"=0, "source"=""} ("error out") w171 w197 w201] -> w127
          tunnel: w126 -> [_ w170 w193 w203]
          tunnel: w125 -> [w132 _ w191 w200]
          tunnel: [w132 w165 w191 w200] -> w124
          tunnel: [w135 enum16{"Close", "Record", "Open", "Idel"}."Record" w187 enum16{"Close", "Record", "Open", "Idel"}."Idel"] -> w123
          frame "Idel", Default {
            n120 = local read "Save"() -> (w136:bool)
            n121 = Select(t=enum16{"Close", "Record", "Open", "Idel"}."Open", s=w136, f=enum16{"Close", "Record", "Open", "Idel"}."Idel") -> (s? t:f=w135:enum16{"Close", "Record", "Open", "Idel"})
          }
          frame "Open" {
            n122 = shared-variable "PXIe-8135\\SharedVariables.lvlib\\Record?"() -> ()  [unwired: 1 in, 2 out]
            n123 = local read "Motor Tuning Param"() -> (w150:T1)
            n124 = Unbundle By Name(w150) -> ("PID Param.GainSchedules"=w149:T10)
            n125 = Index Array(array=w149, index=0) -> (element=w147:T11)
            n126 = Unbundle By Name(w147) -> ("PID gains"=w145:cluster{"Kc":dbl, "Ti":dbl, "Td":dbl})
            n127 = Get Date/Time In Seconds() -> (seconds since 1Jan1904=w141:timestamp)
            n128 = local read "PlannedTension"() -> (w159:dbl[])
            n129 = local read "Actual Tensions"() -> (w156:dbl[])
            n130 = local read "AO_Value"() -> (w157:sgl[])
            n131 = local read "Motor#"() -> (w148:enum16{"1", "2", "3", "4", "5", "6", "7", "8"})
            n132 = Cluster To Array(cluster=w145) -> (array=w146:dbl[])
            n133 = Format Date/Time String(seconds (now)=w141) -> (date/time string=w140:string)  [unwired: 2 in]
            n134 = local read "Save"() -> (w139:bool)
            n135 = Index Array(array=w159, index=w148) -> (element=w158:dbl)
            n136 = Index Array(array=w156, index=w148) -> (element=w155:dbl)
            n137 = Index Array(array=w157, index=w148) -> (element=w169:sgl)
            n138 = Concatenate Strings(w140, " Kc\tTi\tTu\n") -> (w142:string)
            n139 = Boolean To (0,1)(Boolean=w139) -> (0, 1=w138:i16)
            n140 = Array To Spreadsheet String(array=w146, 3:"%.8f" ("format string")) -> (spreadsheet string=w154:string)  [unwired: 1 in]
            n141 = Concatenate Strings(w142, w154, "Time\tSetPoint\tForce(N)\tVO\n" ("Header")) -> (w151:string)
            n142 = Build Array(0.0 ("element"), w158, w155, w169, w138) -> (w168:dbl[])
            n143 = Build Path(base path=path "c:/", name or relative path="ProjectFolder") -> (appended path=w162:path)
            n144 = call "DataLogger_OpenFile.vi"("base path (C:\\CAlex\\)"=w162, "error in (no error)"=w170, "Header"=w151, "File Name"="File Name", "Data Logger in"=w175) -> ("error out"=w172:errorcluster, "Data Logger out"=w173:refnum<class "Data Logger.lvclass">)  [unwired: 5 in]
            n145 = call "Array2Line.vi"("Data"=w168) -> ("String"=w167:string)  [unwired: 10 in]
            n146 = call "DataLogger_WriteData.vi"("error in (no error)"=w172, "New line"=w167, "Data Logger in"=w173) -> ("error out"=w171:errorcluster, "Data Logger out"=w174:refnum<class "Data Logger.lvclass">)  [unwired: 7 in]
            n147 = Tick Count (ms)() -> (millisecond timer value=w165:u32)
          }
          frame "Record" {
            n148 = Tick Count (ms)() -> (millisecond timer value=w192:u32)
            n149 = Subtract(x=w192, y=w191) -> (x-y=w186:dbl)
            n150 = local read "Save"() -> (w176:bool)
            n151 = local read "PlannedTension"() -> (w184:dbl[])
            n152 = local read "Actual Tensions"() -> (w182:dbl[])
            n153 = local read "AO_Value"() -> (w183:sgl[])
            n154 = expression code="x/1000"(w186) -> (w185:dbl)
            n155 = local read "Motor#"() -> (w181:enum16{"1", "2", "3", "4", "5", "6", "7", "8"})
            n156 = Boolean To (0,1)(Boolean=w176) -> (0, 1=w177:i16)
            n157 = Index Array(array=w184, index=w181) -> (element=w180:dbl)
            n158 = Index Array(array=w182, index=w181) -> (element=w179:dbl)
            n159 = Index Array(array=w183, index=w181) -> (element=w178:sgl)
            n160 = Build Array(w185, w180, w179, w178, w177) -> (w196:dbl[])
            n161 = call "Array2Line.vi"("Data"=w196) -> ("String"=w195:string)  [unwired: 10 in]
            n162 = call "DataLogger_WriteData.vi"("error in (no error)"=w193, "New line"=w195, "Data Logger in"=w194) -> ("error out"=w197:errorcluster, "Data Logger out"=w198:refnum<class "Data Logger.lvclass">)  [unwired: 7 in]
            n163 = local read "Save"() -> (w190:bool)
            n164 = Select(t=enum16{"Close", "Record", "Open", "Idel"}."Record", s=w190, f=enum16{"Close", "Record", "Open", "Idel"}."Close") -> (s? t:f=w187:enum16{"Close", "Record", "Open", "Idel"})
          }
          frame "Close" {
            n165 = call "DataLogger_CloseFile.vi"("error in (no error)"=w203, "Data Logger in"=w204) -> ("error out"=w201:errorcluster, "Data Logger out"=w202:refnum<class "Data Logger.lvclass">)  [unwired: 8 in]
          }
        }
        n166 = local read "stop"() -> (w122:bool)
        n167 = node-c288() -> ()  [unwired: 1 in, 1 out]
      }
      n168 = node-c288(w69) -> ()  [unwired: 1 out]
      n169 = disable-structure shown="Enabled" {
        frame Enabled {
          n170 = node-c288() -> (w210:T6)  [unwired: 4 in]
          n171 = timed-loop {
            timing: w210 -> [_]
            timing-out: [_] -> w209
            stop <- w222 stop-if-true
            n172 = node-c288() -> ()  [unwired: 1 in, 1 out]
            n173 = feedback #2() -> (w228:dbl)  [unwired: 1 in]
            n174 = feedback-in #2("phase") -> ()
            n175 = Subtract(x="phase", y=w228) -> (x-y=w227:dbl)
            n176 = Add(x="offset", y="amplitude") -> (x+y=w216:dbl)
            n177 = feedback #3() -> (w226:dbl)  [unwired: 1 in]
            n178 = Add(x=w227, y=w226) -> (x+y=w232:dbl)
            n179 = call <vilib>:"Basic Function Generator.vi"("offset"=w216, "reset signal"="reset signal", "sampling info"=cluster{"Fs":dbl, "#s":dbl} {"Fs"=1000.0, "#s"=1.0}, "signal type"="signal type", "phase"=w232, "amplitude"="amplitude", "frequency"="frequency") -> ("phase out"=w225:dbl, "signal out"=w223:waveform(dbl))  [unwired: 2 in, 1 out]
            n180 = feedback-in #3(w225) -> ()
            n181 = Unbundle By Name(w223) -> ("Y"=w220:dbl[])
            n182 = Reverse 1D Array(array=w220) -> (reversed array=w219:dbl[])
            n183 = Index Array(array=w219) -> (element=w214:dbl)  [unwired: 1 in]
            n184 = In Range and Coerce(upper limit=100.0, x=w214, lower limit=0.0) -> (coerced(x)=w212:dbl)  [unwired: 1 out]
            "funcgen" <- w212
            n185 = Bundle("upper limit"=w212) -> (→"Signal Command":cluster{"upper limit":dbl})  [unwired: 1 in]
            n186 = local read "stop"() -> (w222:bool)
            n187 = node-c288() -> ()  [unwired: 1 in, 1 out]
          }
          n188 = node-c288(w209) -> ()  [unwired: 1 out]
        }
        frame Disabled {
          n189 = local read "Motor#"() -> ()  [unwired: 1 out]
        }
      }
      n190 = node-c288(w79) -> ()  [unwired: 1 out]
      n191 = node-c288(w91) -> (w64:errorcluster)
      n192 = case shown="No Error" w64 {
        frame No Error {
          n193 = local write "stop"(TRUE) -> ()
        }
        frame Error {
        }
      }
      n194 = property class="MotorCtrl"(reference=w66) -> ("PropertyNode:MotorQuantity"=w65:i32)  [unwired: 1 in, 2 out]
      n195 = call <vilib>:"DAQmx Stop Task.vi"("task/channels in"=w75) -> ("task out"=w74:refnum<k21>, "error out"=w71:errorcluster)  [unwired: 13 in]
      n196 = call <vilib>:"DAQmx Clear Task.vi"("task in"=w74, "error in"=w71) -> ()  [unwired: 13 in, 1 out]
      n197 = Initialize Array(0.0 ("element"), w65) -> (w83:dbl[])
      n198 = Initialize Array(FALSE, w65) -> (w82:bool[])
      n199 = call <vilib>:"DAQmx Stop Task.vi"("task/channels in"=w59) -> ("task out"=w61:refnum<k21>, "error out"=w60:errorcluster)  [unwired: 13 in]
      n200 = for {
        tunnel: w71 -> [w121]
        tunnel: w72 -> [w120] mode=indexing
        n201 = call <vilib>:"DAQmx Clear Task.vi"("task in"=w120, "error in"=w121) -> ()  [unwired: 13 in, 1 out]
      }
      n202 = xnode "Read/Write Control"("FPGA VI Reference In"=w67, "AmpCmd"=w83, "Enable"=w82, "EnableMaster"=FALSE) -> ("FPGA VI Reference Out"=w87:refnum<k20>, "error out"=w86:errorcluster)  [unwired: 1 in]
      n203 = call <vilib>:"DAQmx Clear Task.vi"("task in"=w61, "error in"=w60) -> ()  [unwired: 13 in, 1 out]
      n204 = xnode "Close FPGA VI Reference"("FPGA VI Reference In"=w87, "error in"=w86) -> ()  [unwired: 1 out]
    }
  }
